vi "Inititalize.vi"(0 "Sift Client in":refnum<class "Sift Client.lvclass">, 5 "API URL":string, 7 "API Key":string, 9 "Organization ID":string, 11 "error in (no error)":errorcluster, 12 "Sift Proxy Address":string="localhost:10010", 13 "Test Mode":bool) -> (4 "Sift Client out":refnum<class "Sift Client.lvclass">, 15 "error out":errorcluster)   [LabVIEW 2024, in "Sift Client.lvlib" / "Sift Client.lvclass"]
doc: "Initializes the Sift Client.\n\nSee https://docs.siftstack.com/docs/api/authentication for more information.\n\nSift Proxy address can be overidden if you want to run it on a different port."
uses:
  Sift Client.lvclass
  Private/Typedefs/Sample.ctl
  Private/Typedefs/Timestamp.ctl
  Private/Testing/Mock REST Client/Mock REST Client.lvclass
  C:/Program Files (x86)/National Instruments/LabVIEW 2024/vi.lib/addons/_JKI.lib/REST Client/classes/REST Client/REST Client.lvclass
  Sift Client.lvclass/Sift Client.ctl
  <vilib>/addons/_JKI.lib/REST Client/classes/REST Client/REST Client.lvclass
  Sift Client.lvlib
panel:
  in  "Sample":T1
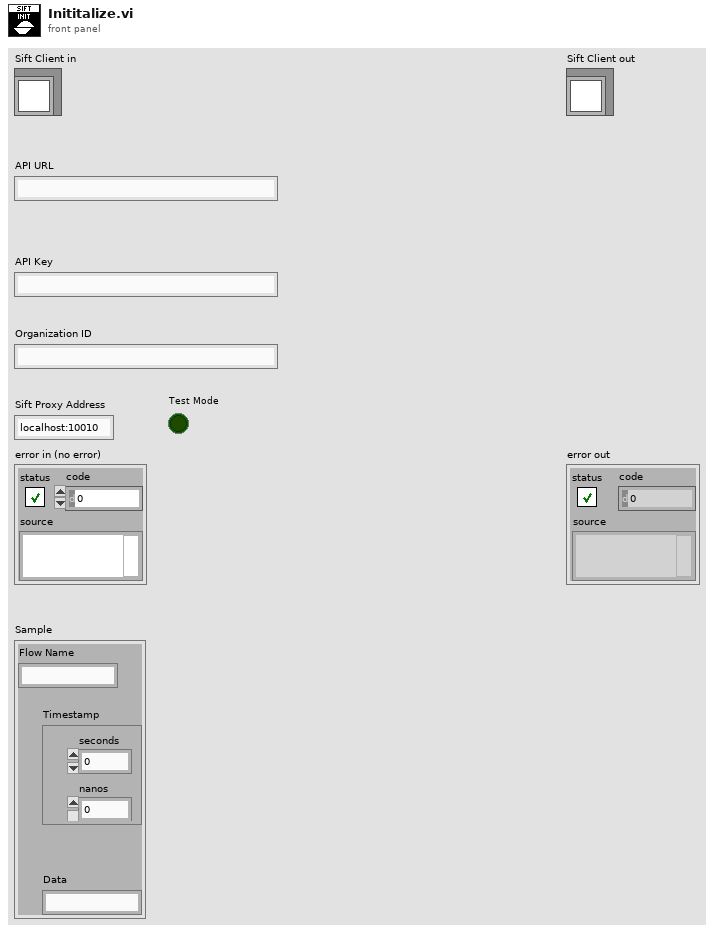
[diagram p1: front panel]
types:
  T1 = typedef "Sift Client.lvlib/Sample.ctl" = cluster{"Flow Name":string, "Timestamp":T2, "Data":string}
  T2 = typedef "Sift Client.lvlib/Timestamp.ctl" = cluster{"seconds":i64, "nanos":i32}
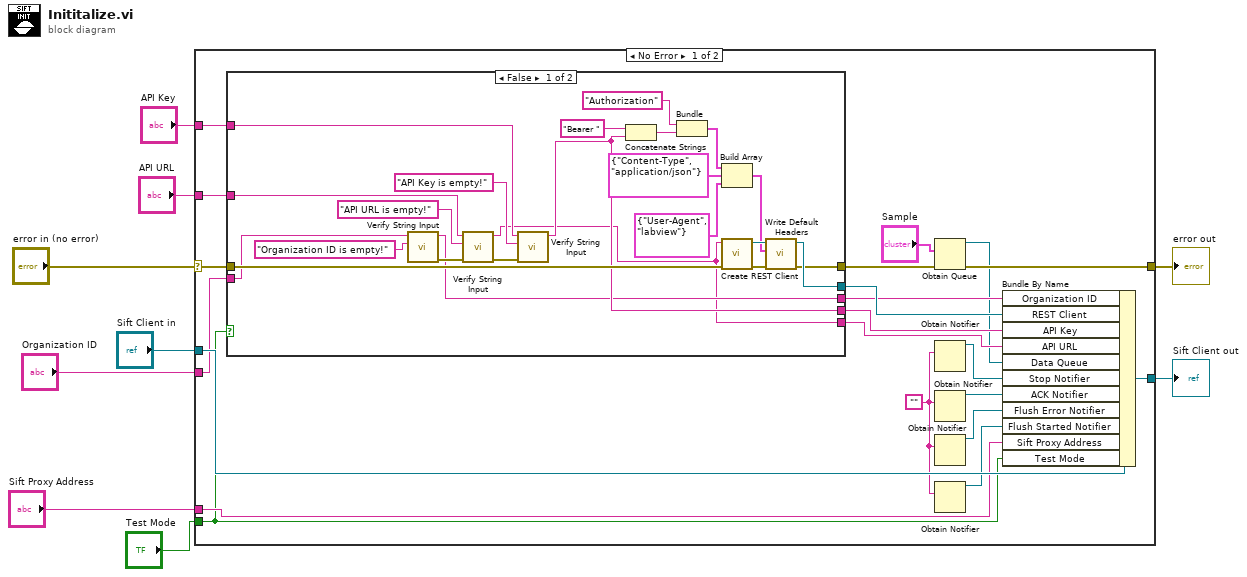
[diagram p0: block diagram]
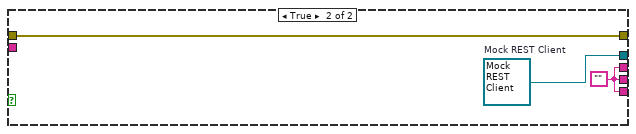
[diagram p2: hidden frame]
diagram:
  n1 = case shown="No Error" "error in (no error)" {
    selector: "error in (no error)" -> [w30 w58]
    tunnel: [w29 w57] -> w7
    tunnel: "Sift Client in" -> [w28 w57]
    tunnel: "API Key" -> [w19 _]
    tunnel: "API URL" -> [w17 _]
    tunnel: "Organization ID" -> [w16 _]
    tunnel: [w26 w58] -> w3
    tunnel: "Test Mode" -> [w10 _]
    tunnel: "Sift Proxy Address" -> [w14 _]
    frame No Error {
      w11 = ""
      n2 = case shown="False" w10 {
        tunnel: w30 -> [w53 w56]
        tunnel: [w50 w55] -> w27
        tunnel: [w32 w54] -> w20
        tunnel: [w49 w56] -> w25
        tunnel: w19 -> [w42 _]
        tunnel: [w41 w54] -> w18
        tunnel: w17 -> [w37 _]
        tunnel: w16 -> [w35 _]
        tunnel: [w33 w54] -> w15
        frame False {
          n3 = call "Verify String Input.vi"("Error Message"="Organization ID is empty!", "Input"=w35) -> ("error out"=w39:errorcluster, "Output"=w33:string)  [unwired: 8 in]
          n4 = call "Verify String Input.vi"("error in (no error)"=w39, "Error Message"="API URL is empty!", "Input"=w37) -> ("error out"=w34:errorcluster, "Output"=w32:string)  [unwired: 7 in]
          n5 = call "Verify String Input.vi"("error in (no error)"=w34, "Error Message"="API Key is empty!", "Input"=w42) -> ("Output"=w41:string)  [unwired: 7 in, 1 out]
          n6 = Concatenate Strings("Bearer ", w41) -> (w44:string)
          n7 = Bundle("Authorization", w44) -> (w46:cluster{string, string})  [unwired: 1 in]
          n8 = Build Array(w46, cluster{string, string} {"Content-Type", "application/json"}, cluster{string, string} {"User-Agent", "labview"}) -> (w48:cluster{string, string}[])
          n9 = call <vilib>:"Create REST Client.vi"("error in (no error)"=w53, "Base URL"=w32) -> ("error out"=w51:errorcluster, "REST Client out"=w52:refnum<class "REST Client.lvclass">)  [unwired: 8 in]
          n10 = call-dynamic "Write Default Headers.vi"("error in (no error)"=w51, "Headers"=w48, "REST Client in"=w52) -> ("error out"=w49:errorcluster, "REST Client out"=w50:refnum<class "REST Client.lvclass">)  [unwired: 7 in]
        }
        frame True {
          w54 = ""
          w55 = refnum<class "Mock REST Client.lvclass"> refnum  # Mock REST Client
        }
      }
      n11 = Obtain Queue(element data type="Sample", error in (no error)=w25) -> (queue out=w12:refnum<queue>, error out=w26:errorcluster)  [unwired: 3 in, 1 out]
      n12 = Obtain Notifier(notification data type=w11) -> (notifier out=w24:refnum<notifier>)  [unwired: 3 in, 2 out]
      n13 = Obtain Notifier(notification data type=w11) -> (notifier out=w23:refnum<notifier>)  [unwired: 3 in, 2 out]
      n14 = Obtain Notifier(notification data type=w11) -> (notifier out=w22:refnum<notifier>)  [unwired: 3 in, 2 out]
      n15 = Obtain Notifier(notification data type=w11) -> (notifier out=w21:refnum<notifier>)  [unwired: 3 in, 2 out]
      n16 = Bundle By Name(cluster=w28, "Organization ID"=w15, "REST Client"=w27, "API Key"=w18, "API URL"=w20, "Data Queue"=w12, "Stop Notifier"=w24, "ACK Notifier"=w23, "Flush Error Notifier"=w22, "Flush Started Notifier"=w21, "Sift Proxy Address"=w14, "Test Mode"=w10) -> (w29:refnum<class "Sift Client.lvclass">)
    }
    frame Error {
    }
  }
  "error out" <- w3
  "Sift Client out" <- w7
